vi "Finish.vi"   [LabVIEW 2012]
doc: "This VI is called just before exiting. It is expected to close I/O refnum, save collected data, etc."
uses:
  <vilib>/Rock Robotics/WPI/Joystick/WPI_JoystickGetSetRefNum.vi
  <vilib>/Rock Robotics/WPI/RobotDrive/WPI_RobotDriveGetSetRefNum.vi
types:
  T1 = typedef "WPI_EncoderDevRef.ctl" = cluster{"DevStatus":errorcluster, "EncoderIndex":T2, "CounterIndex":T3, "DistancePerCount":dbl, "Decoding Type":T4}
  T2 = typedef "FPGA_EncoderIdx.ctl" = enum8{"Enc 0", "Enc 1", "Enc 2", "Enc 3", "Invalid"}
  T3 = typedef "FPGA_CounterCtrSystemIndex.ctl" = enum8{"Ctr 0", "Ctr 1", "Ctr 2", "Ctr 3", "Ctr 4", "Ctr 5", "Ctr 6", "Ctr 7", "Invalid"}
  T4 = typedef "WPI_EncoderType.ctl" = enum16{"1x", "2x", "4x"}
  T5 = typedef "WPI_AnalogChannelDevRef.ctl" = cluster{"DevStatus":errorcluster, "Analog Module":T6, "Analog Channel":T7}
  T6 = typedef "FPGA_TypedefAnalogModule.ctl" = enum16{"Analog Module 1", "Analog Module 2"}
  T7 = typedef "FPGA_AIChannel.ctl" = enum8{"AI 1", "AI 2", "AI 3", "AI 4", "AI 5", "AI 6", "AI 7", "AI 8", "Invalid"}
  T8 = typedef "WPI_SolenoidDevRef.ctl" = cluster{"DevStatus":errorcluster, "Solenoid Module":T9, "Forward Solenoid Channel":T10, "Reverse Solenoid Channel":T10}
  T9 = typedef "FPGA_TypedefSolenoidModule.ctl" = enum16{"Solenoid Module 1", "Solenoid Module 2"}
  T10 = typedef "WPI_SolenoidChannel.ctl" = enum8{"Solenoid 1", "Solenoid 2", "Solenoid 3", "Solenoid 4", "Solenoid 5", "Solenoid 6", "Solenoid 7", "Solenoid 8", "Invalid"}
  T11 = typedef "WPI_MotorControlDeviceRef.ctl" = cluster{"DeviceStatus":errorcluster, "Type":enum16{"PWM", "CAN"}, "PWM":cluster{"Digital Module":T12, "PWM Channel":T13, "DeadBand":T14}, "CAN":cluster{"Device Number":u8, "Control Mode":T15, "Semaphore":T16, "Max Vout":dbl}, "Invert":bool, "TransformRef":T17, "InvTransformRef":T17}
  T12 = typedef "FPGA_TypedefDigitalModule.ctl" = enum16{"Digital Module 1", "Digital Module 2"}
  T13 = typedef "FPGA_DIOPWMChannel.ctl" = enum8{"PWM 1", "PWM 2", "PWM 3", "PWM 4", "PWM 5", "PWM 6", "PWM 7", "PWM 8", "PWM 9", "PWM 10", "Invalid"}
  T14 = typedef "WPI_PWMDeadband.ctl" = cluster{"Name":string, "maxPositivePwm":i32, "minPositivePwm":i32, "centerPwm":i32, "maxNegativePwm":i32, "minNegativePwm":i32, "angularRange":u16}
  T15 = typedef "WPI_CANJaguar_ControlMode.ctl" = enum8{"Percent VBus", "Current", "Speed", "Position", "Voltage"}
  T16 = typedef "Semaphore RefNum" = refnum<k1>
  T17 = typedef "WPI_PWMTransform_ConPane.ctl" = refnum<vi>
  T18 = typedef "WPI_CameraDevRef.ctl" = cluster{"Camera Address":string, "CameraStatus":errorcluster, "Acquire Image Notifier":refnum<notifier>}
  T19 = typedef "WPI_ServoDeviceRef.ctl" = cluster{"DeviceStatus":errorcluster, "Digital Module":T12, "PWM Channel":T13, "DeadBand":T14}
  T20 = typedef "WPI_RelayDevRef.ctl" = cluster{"DevStatus":errorcluster, "Relay Channel":T21, "Digital Module":T12, "Relay Direction":T22}
  T21 = typedef "FPGA_DIORelayChannel.ctl" = enum8{"Relay 1", "Relay 2", "Relay 3", "Relay 4", "Relay 5", "Relay 6", "Relay 7", "Relay 8", "Invalid"}
  T22 = typedef "WPI_RelayDirection.ctl" = enum16{"Both directions", "Forward only", "Reverse only"}
  T23 = typedef "WPI_JoystickDevRef.ctl" = cluster{"Device":T24}
  T24 = typedef "WPI_JoystickDeviceEnum.ctl" = enum16{"USB 1", "USB 2", "USB 3", "USB 4", "Kinect 1", "Kinect 2"}
  T25 = typedef "WPI_RobotDriveDevRef.ctl" = cluster{"DevStatus":errorcluster, "Motors[]":T11[], "Square Inputs":bool, "Max Output":dbl, "Isochronous":bool}
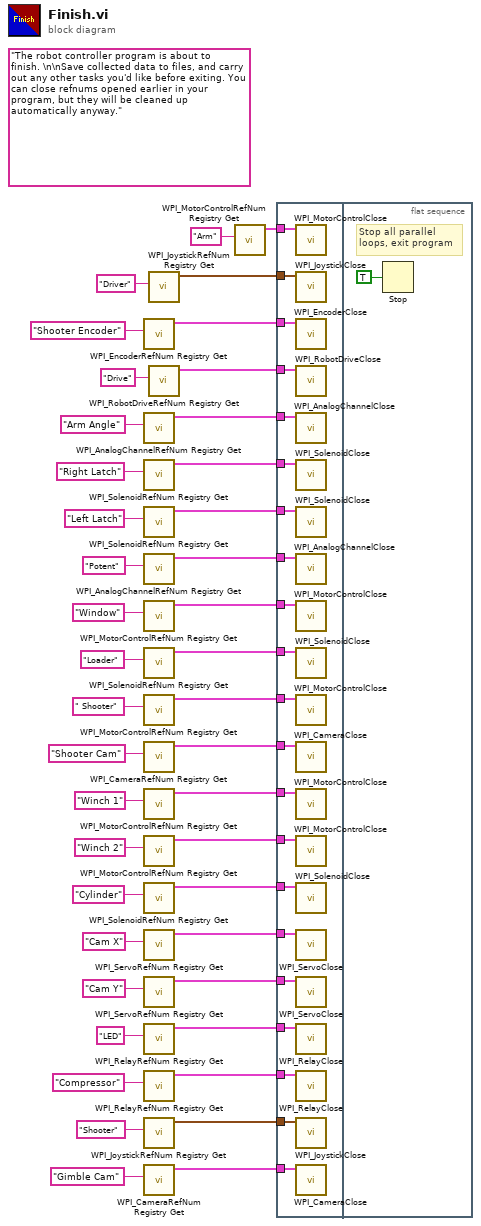
[diagram p0: block diagram]
diagram:
  (unwired) "The robot controller program is about to finish. \n\nSave collected data to files, and carry out any other tasks you'd like before exiting. You can close refnums opened earlier in your program, but they will be cleaned up automatically anyway."
  n1 = call <vilib>:"WPI_EncoderRefNum Registry Get.vi"("refnum name"="Shooter Encoder") -> ("EncoderDevRef"=w20:T1)  [unwired: 9 in, 1 out]
  n2 = call <vilib>:"WPI_AnalogChannelRefNum Registry Get.vi"("refnum name"="Arm Angle") -> ("AIDeviceRef"=w1:T5)  [unwired: 9 in, 1 out]
  n3 = call <vilib>:"WPI_SolenoidRefNum Registry Get.vi"("refnum name"="Right Latch") -> ("SolenoidDevRef"=w3:T8)  [unwired: 9 in, 1 out]
  n4 = call <vilib>:"WPI_SolenoidRefNum Registry Get.vi"("refnum name"="Left Latch") -> ("SolenoidDevRef"=w4:T8)  [unwired: 9 in, 1 out]
  n5 = call <vilib>:"WPI_AnalogChannelRefNum Registry Get.vi"("refnum name"="Potent") -> ("AIDeviceRef"=w7:T5)  [unwired: 9 in, 1 out]
  n6 = call <vilib>:"WPI_MotorControlRefNum Registry Get.vi"("refnum name"="Window") -> ("MotorControlDevRef"=w9:T11)  [unwired: 9 in, 1 out]
  n7 = call <vilib>:"WPI_SolenoidRefNum Registry Get.vi"("refnum name"="Loader") -> ("SolenoidDevRef"=w12:T8)  [unwired: 9 in, 1 out]
  n8 = call <vilib>:"WPI_MotorControlRefNum Registry Get.vi"("refnum name"=" Shooter") -> ("MotorControlDevRef"=w13:T11)  [unwired: 9 in, 1 out]
  n9 = call <vilib>:"WPI_CameraRefNum Registry Get.vi"("refnum name"="Shooter Cam") -> ("CameraDevRef"=w17:T18)  [unwired: 1 in, 9 out]
  n10 = call <vilib>:"WPI_MotorControlRefNum Registry Get.vi"("refnum name"="Winch 1") -> ("MotorControlDevRef"=w23:T11)  [unwired: 9 in, 1 out]
  n11 = call <vilib>:"WPI_MotorControlRefNum Registry Get.vi"("refnum name"="Winch 2") -> ("MotorControlDevRef"=w24:T11)  [unwired: 9 in, 1 out]
  n12 = call <vilib>:"WPI_SolenoidRefNum Registry Get.vi"("refnum name"="Cylinder") -> ("SolenoidDevRef"=w26:T8)  [unwired: 9 in, 1 out]
  n13 = call <vilib>:"WPI_ServoRefNum Registry Get.vi"("refnum name"="Cam X") -> ("ServoDeviceRef"=w29:T19)  [unwired: 9 in, 1 out]
  n14 = call <vilib>:"WPI_ServoRefNum Registry Get.vi"("refnum name"="Cam Y") -> ("ServoDeviceRef"=w30:T19)  [unwired: 9 in, 1 out]
  n15 = call <vilib>:"WPI_RelayRefNum Registry Get.vi"("refnum name"="LED") -> ("RelayDevRef"=w33:T20)  [unwired: 9 in, 1 out]
  n16 = call <vilib>:"WPI_RelayRefNum Registry Get.vi"("refnum name"="Compressor") -> ("RelayDevRef"=w34:T20)  [unwired: 9 in, 1 out]
  n17 = call <vilib>:"WPI_JoystickRefNum Registry Get.vi"("refnum name"="Shooter") -> ("JoystickDevRef"=w35:T23)  [unwired: 1 in, 9 out]
  n18 = call <vilib>:"WPI_CameraRefNum Registry Get.vi"("refnum name"="Gimble Cam") -> ("CameraDevRef"=w38:T18)  [unwired: 1 in, 9 out]
  n19 = call <vilib>:"WPI_JoystickRefNum Registry Get.vi"("refnum name"="Driver") -> ("JoystickDevRef"=w39:T23)  [unwired: 1 in, 9 out]
  n20 = call <vilib>:"WPI_RobotDriveRefNum Registry Get.vi"("refnum name"="Drive") -> ("RobotDriveDevRef"=w40:T25)  [unwired: 1 in, 9 out]
  n21 = call <vilib>:"WPI_MotorControlRefNum Registry Get.vi"("refnum name"="Arm") -> ("MotorControlDevRef"=w14:T11)  [unwired: 9 in, 1 out]
  n22 = flat-sequence {
    tunnel: w40 -> [w63]
    tunnel: w39 -> [w62]
    tunnel: w38 -> [w61]
    tunnel: w35 -> [w60]
    tunnel: w34 -> [w59]
    tunnel: w33 -> [w58]
    tunnel: w30 -> [w57]
    tunnel: w29 -> [w56]
    tunnel: w26 -> [w55]
    tunnel: w24 -> [w54]
    tunnel: w23 -> [w53]
    tunnel: w20 -> [w52]
    tunnel: w17 -> [w51]
    tunnel: w14 -> [w50]
    tunnel: w13 -> [w49]
    tunnel: w12 -> [w48]
    tunnel: w9 -> [w47]
    tunnel: w7 -> [w46]
    tunnel: w4 -> [w45]
    tunnel: w3 -> [w44]
    tunnel: w1 -> [w43]
    frame #0 {
      n23 = call <vilib>:"WPI_MotorControlClose.vi"("MotorControlDevRef"=w50) -> ()  [unwired: 10 in, 1 out]
      n24 = call <vilib>:"WPI_JoystickClose.vi"("JoystickDevRef"=w62) -> ()  [unwired: 11 out]
      n25 = call <vilib>:"WPI_EncoderClose.vi"("EncoderDevRef"=w52) -> ()  [unwired: 10 in, 1 out]
      n26 = call <vilib>:"WPI_RobotDriveClose.vi"("RobotDriveDevRef"=w63) -> ()  [unwired: 1 in, 10 out]
      n27 = call <vilib>:"WPI_AnalogChannelClose.vi"("AIDeviceRef"=w43) -> ()  [unwired: 10 in, 1 out]
      n28 = call <vilib>:"WPI_SolenoidClose.vi"("SolenoidDevRef"=w44) -> ()  [unwired: 10 in, 1 out]
      n29 = call <vilib>:"WPI_SolenoidClose.vi"("SolenoidDevRef"=w45) -> ()  [unwired: 10 in, 1 out]
      n30 = call <vilib>:"WPI_AnalogChannelClose.vi"("AIDeviceRef"=w46) -> ()  [unwired: 10 in, 1 out]
      n31 = call <vilib>:"WPI_MotorControlClose.vi"("MotorControlDevRef"=w47) -> ()  [unwired: 10 in, 1 out]
      n32 = call <vilib>:"WPI_SolenoidClose.vi"("SolenoidDevRef"=w48) -> ()  [unwired: 10 in, 1 out]
      n33 = call <vilib>:"WPI_MotorControlClose.vi"("MotorControlDevRef"=w49) -> ()  [unwired: 10 in, 1 out]
      n34 = call <vilib>:"WPI_CameraClose.vi"("CameraDevRef"=w51) -> ()  [unwired: 1 in, 10 out]
      n35 = call <vilib>:"WPI_MotorControlClose.vi"("MotorControlDevRef"=w53) -> ()  [unwired: 10 in, 1 out]
      n36 = call <vilib>:"WPI_MotorControlClose.vi"("MotorControlDevRef"=w54) -> ()  [unwired: 10 in, 1 out]
      n37 = call <vilib>:"WPI_SolenoidClose.vi"("SolenoidDevRef"=w55) -> ()  [unwired: 10 in, 1 out]
      n38 = call <vilib>:"WPI_ServoClose.vi"("MotorControlDevRef"=w56) -> ()  [unwired: 10 in, 1 out]
      n39 = call <vilib>:"WPI_ServoClose.vi"("MotorControlDevRef"=w57) -> ()  [unwired: 10 in, 1 out]
      n40 = call <vilib>:"WPI_RelayClose.vi"("RelayDevRef"=w58) -> ()  [unwired: 10 in, 1 out]
      n41 = call <vilib>:"WPI_RelayClose.vi"("RelayDevRef"=w59) -> ()  [unwired: 10 in, 1 out]
      n42 = call <vilib>:"WPI_JoystickClose.vi"("JoystickDevRef"=w60) -> ()  [unwired: 11 out]
      n43 = call <vilib>:"WPI_CameraClose.vi"("CameraDevRef"=w61) -> ()  [unwired: 1 in, 10 out]
    }
    frame #1 {
      # "Stop all parallel\nloops, exit program"
      n44 = Stop(stop? (T)=TRUE ("Quit")) -> ()
    }
  }
